vi "sv_Verify Resampled Signal (OMP).vi"(0 "resampled signal":cluster{"r0":dbl, "dr":dbl, "Y":dbl[]}[](array[cluster]) {"r0" format="%.2p"; "dr" format="%.2p"; "Y" format="%.2f"}, 1 "reset in (T)":bool=TRUE, 7 "orders to compute (1.0)":dbl[](array[numeric])=[1.0] format="%.2f", 9 "bandwidth [order]":dbl=1.0 format="%.2f", 11 "error in (no error)":errorcluster) -> (3 "reset out (T)":bool=TRUE, 4 "resampled signal out":cluster{"r0":dbl, "dr":dbl, "Y":dbl[]}[](array[cluster]), 8 "orders to compute (1.0) out":dbl[](array[numeric])=[1.0] format="%.2f", 10 "bandwidth [order] out":dbl=1.0 format="%.2f", 15 "error out":errorcluster)   [LabVIEW 2017, in "SoundVib_ContSweptSine.lvlib"]
uses:
  <vilib>/addons/Sound and Vibration/svt_Continuous Swept Sine/SoundVib_ContSweptSine.lvlib
  <vilib>/addons/Sound and Vibration/Order Analysis/Resample Order Tracking/SubVIs/OAT Verify Resampled Signal (Multi Channels).vi
  <vilib>/addons/Sound and Vibration/Order Analysis/Resample Order Tracking/SoundVib_Resampling.lvlib
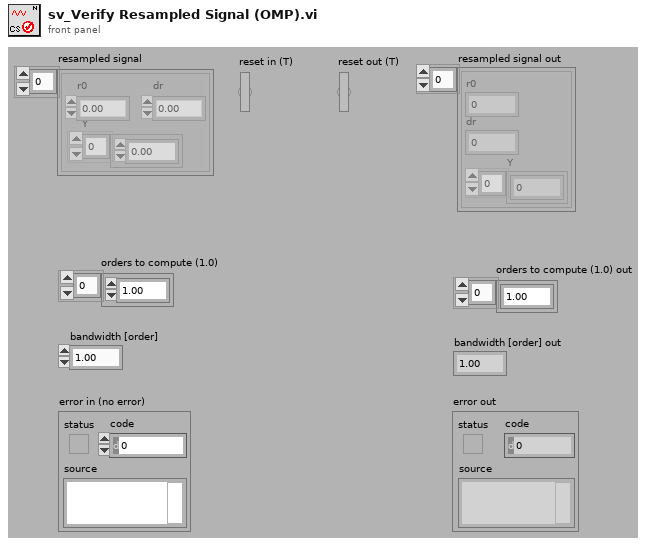
[diagram p1: front panel]
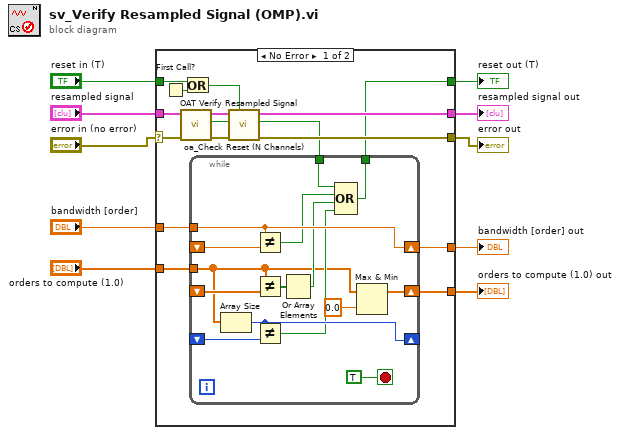
[diagram p0: block diagram]
diagram:
  n1 = case shown="No Error" "error in (no error)" {
    selector: "error in (no error)" -> [w21 w44]
    tunnel: [w19 w44] -> w10
    tunnel: [w20 w45] -> w9
    tunnel: "reset in (T)" -> [w26 w46]
    tunnel: [w11 w46] -> w7
    tunnel: "orders to compute (1.0)" -> [w16 w43]
    tunnel: "bandwidth [order]" -> [w15 w42]
    tunnel: [w13 w43] -> w4
    tunnel: [w14 w42] -> w3
    tunnel: "resampled signal" -> [w22 w45]
    frame No Error {
      n2 = First Call?() -> (First Call?: T/F=w25:bool)
      n3 = call-poly <vilib>:"OAT Verify Resampled Signal.vi"("error in (no error)"=w21, "resampled signal"=w22) -> ("error out"=w23:errorcluster, "empty signal"=w12:bool, "resampled signal out"=w24:cluster{"r0":dbl, "dr":dbl, "Y":dbl[]}[])  [unwired: 7 out]
      n4 = Or(x=w26, y=w25) -> (x .or. y?=w18:bool)
      n5 = call <vilib>:"oa_Check Reset (N Channels).vi"("reset?"=w18, "error in (no error)"=w23, "empty?"=w12, "resampled signal"=w24) -> ("error out"=w19:errorcluster, "reset?"=w17:bool, "resampled signal out"=w20:cluster{"r0":dbl, "dr":dbl, "Y":dbl[]}[])  [unwired: 5 out]
      n6 = while {
        shift-right: [w39] -> w14
        shift-left: _ -> [w40]
        tunnel: w15 -> [w39]
        tunnel: w16 -> [w30]
        shift-right: [w28] -> w13
        shift-left: _ -> [w38]
        shift-right: [w35] -> _
        shift-left: _ -> [w36]
        tunnel: [w31] -> w11
        tunnel: w17 -> [w27]
        stop <- TRUE stop-if-true
        n7 = Array Size(array=w30) -> (size(s)=w35:i32)
        n8 = Not Equal?(x=w39, y=w40) -> (x != y?=w34:bool)
        n9 = Not Equal?(x=w30, y=w38) -> (x != y?=w37:bool[])
        n10 = Not Equal?(x=w35, y=w36) -> (x != y?=w32:bool)
        n11 = Or Array Elements(Boolean array=w37) -> (logical OR=w33:bool)
        n12 = Compound Arithmetic op=OR(w27, w34, w33, w32) -> (w31:bool)
        n13 = Max & Min(x=w30, y=0.0) -> (max(x,y)=w28:dbl[])  [unwired: 1 out]
      }
    }
    frame Error {
    }
  }
  "error out" <- w10
  "resampled signal out" <- w9
  "reset out (T)" <- w7
  "orders to compute (1.0) out" <- w4
  "bandwidth [order] out" <- w3
